vi "set_relays.vi"(8 "error in (no error)":errorcluster, 9 "card address":u8=1, 10 "boolian array in":bool[](array[boolean]), 11 "VISA Refnum in":refnum<visa-resource-name>) -> (0 "error out":errorcluster, 1 "return string":string, 2 "boolian array out":bool[](array[boolean]), 3 "VISA Refnum out":refnum<visa-resource-name>)   [LabVIEW 2018]
doc: "Command 3 is issued.\nSets all 8 relays of the selected card (card number) to the selected values given in the boolian array"
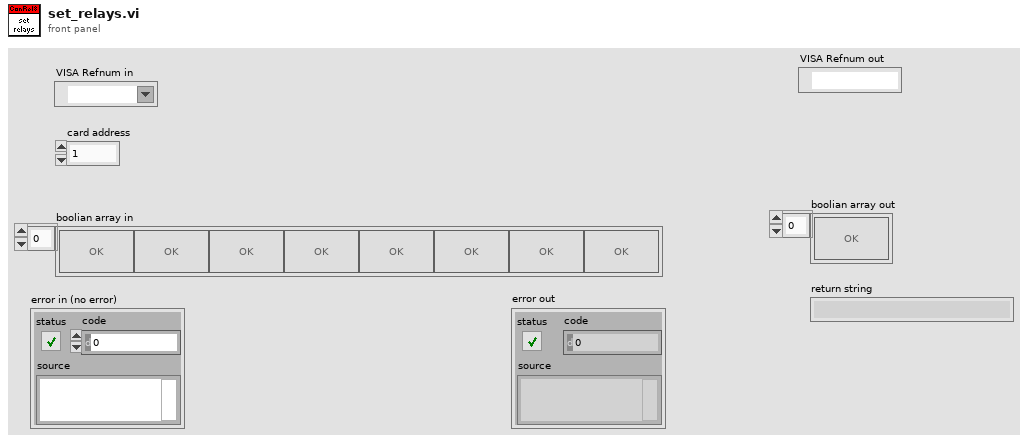
[diagram p1: front panel]
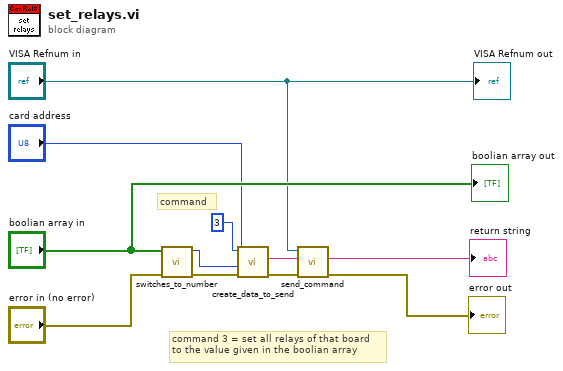
[diagram p0: block diagram]
diagram:
  # "command 3 = set all relays of that board\nto the value given in the boolian array"
  # "command"
  n1 = call "switches_to_number.vi"("error in (no error)"="error in (no error)", "switches"="boolian array in") -> ("error out"=w5:errorcluster, "number"=w7:u8)  [unwired: 4 in]
  n2 = call "create_data_to_send.vi"("error in (no error)"=w5, "data"=w7, "address"="card address", "command"=u8 3) -> ("error out"=w8:errorcluster, "send string"=w11:string)  [unwired: 4 in, 2 out]
  n3 = call "send_command.vi"("error in (no error)"=w8, "command"=w11, "VISA Refnum in"="VISA Refnum in") -> ("error out"=→"error out":errorcluster, "return string"=→"return string":string)  [unwired: 5 in, 2 out]
  "boolian array out" <- "boolian array in"
  "VISA Refnum out" <- "VISA Refnum in"
